vi "setClusterElement.vi"(6 "Value":variant, 7 "Label.Text":string, 8 "error in (no error)":errorcluster, 10 "reference":refnum<vi>, 11 "Experiment in":refnum<class "Experiment.lvclass">) -> (0 "error out":errorcluster, 2 "reference 2":refnum<vi>, 3 "Experiment out":refnum<class "Experiment.lvclass">)   [LabVIEW 2014, in "Experiment.lvclass"]
uses:
  Experiment.lvclass
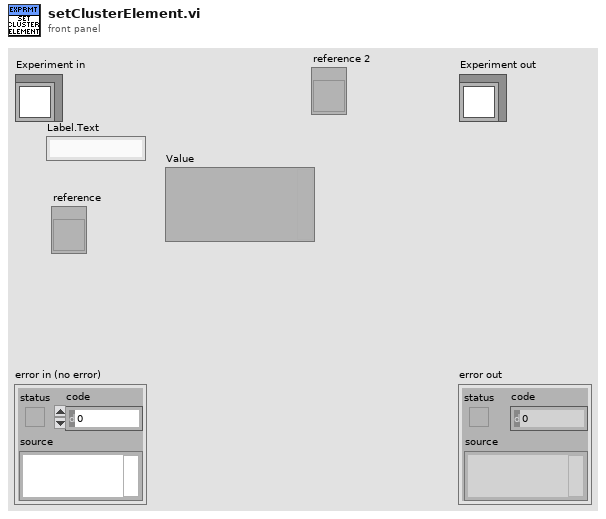
[diagram p1: front panel]
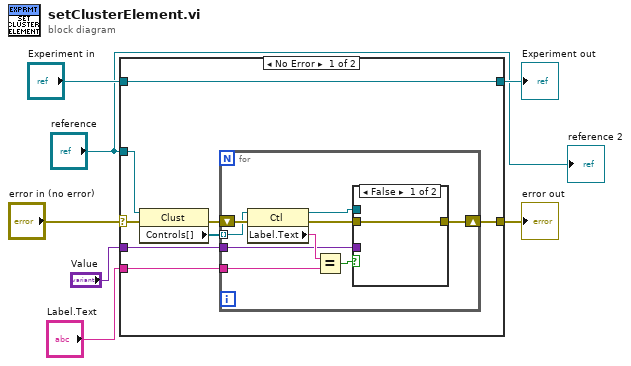
[diagram p0: block diagram]
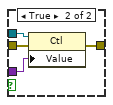
[diagram p2: hidden frame]
diagram:
  n1 = case shown="No Error" "error in (no error)" {
    selector: "error in (no error)" -> [w12 w31]
    tunnel: [w11 w31] -> w6
    tunnel: [w13 w30] -> w4
    tunnel: "Experiment in" -> [w13 w30]
    tunnel: "reference" -> [w10 _]
    tunnel: "Label.Text" -> [w9 _]
    tunnel: "Value" -> [w8 _]
    frame No Error {
      n2 = property class="Clust"(reference=w10, error in=w12) -> (error out=w15:errorcluster, "Controls[]"=w14:refnum<vi>[])  [unwired: 1 out]
      n3 = for {
        shift-right: [w16] -> w11
        shift-left: w15 -> [w24]
        tunnel: w14 -> [w23] mode=indexing
        tunnel: w9 -> [w20]
        tunnel: w8 -> [w17]
        n4 = property class="Ctl"(reference=w23, error in=w24) -> (reference out=w18:refnum<vi>, error out=w22:errorcluster, "Label.Text"=w21:string)
        n5 = Equal?(x=w21, y=w20) -> (x = y?=w19:bool)
        n6 = case shown="False" w19 {
          tunnel: w22 -> [w25 w27]
          tunnel: w18 -> [_ w29]
          tunnel: w17 -> [_ w28]
          tunnel: [w25 w26] -> w16
          frame False {
          }
          frame True {
            n7 = property class="Ctl"(reference=w29, error in=w27, "Value"=w28) -> (error out=w26:errorcluster)  [unwired: 1 out]
          }
        }
      }
    }
    frame Error {
    }
  }
  "error out" <- w6
  "Experiment out" <- w4
  "reference 2" <- "reference"
